vi "canoptstr.vi"(1 "new element/subarray":i32, 2 "index":i32=4, 3 "String 2":string="t20283F0000099CFF0A00\r") -> (0 "String":string)   [LabVIEW 2017]
panel:
  out "String 3":string
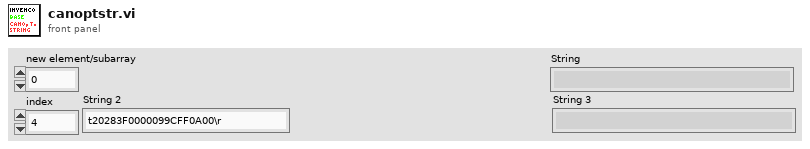
[diagram p1: front panel]
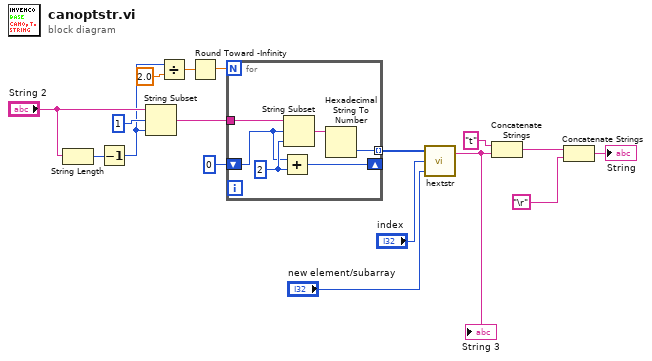
[diagram p0: block diagram]
diagram:
  n1 = String Length(string="String 2") -> (length=w16:i32)
  n2 = Decrement(x=w16) -> (x-1=w11:i32)
  n3 = String Subset(string="String 2", offset (0)=1 ("length (rest)"), length (rest)=w11) -> (substring=w15:string)
  n4 = Divide(x=w11, y=2.0) -> (x/y=w10:dbl)
  n5 = Round Toward -Infinity(1:w10) -> (0:w9:dbl)
  n6 = for {
    N: w9 -> [_]
    tunnel: w15 -> [w23]
    tunnel: [w18] -> w8 mode=indexing
    shift-right: [w21] -> _
    shift-left: 0 ("offset (0)") -> [w20]
    w22 = 2 ("length (rest)")
    n7 = Add(x=w20, y=w22) -> (x+y=w21:i32)
    n8 = String Subset(string=w23, offset (0)=w20, length (rest)=w22) -> (substring=w19:string)
    n9 = Hexadecimal String To Number(string=w19) -> (number=w18:u32)  [unwired: 2 in, 1 out]
  }
  n10 = call "hextstr.vi"("new element/subarray"="new element/subarray", "index"="index", "Array"=w8) -> ("String"=w5:string)  [unwired: 1 out]
  "String 3" <- w5
  n11 = Concatenate Strings("t" ("string"), w5) -> (w3:string)
  n12 = Concatenate Strings(w3, "\r") -> (→"String":string)
